vi "MTS_AutoZPos.vi"(0 "PH Dev":i32, 1 "OFlow Interv [s]":dbl, 2 "Accum Time [s]":dbl, 5 "PI System no.":i32, 11 "error in":errorcluster, 12 "Start Point":T1, 13 "Steps":i32, 14 "Step Width [um]":dbl) -> (4 "New Z":dbl, 6 "Counts":u32[](array[numeric]), 15 "error out":errorcluster)   [LabVIEW 2009]
panel:
  out "FiFo Overrun":bool
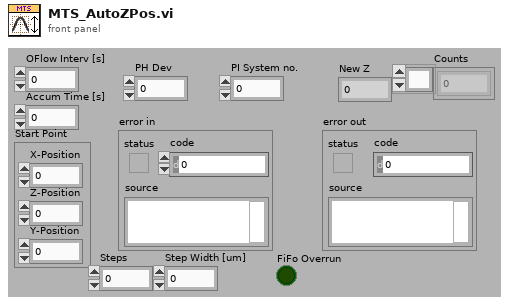
[diagram p1: front panel]
types:
  T1 = cluster{"X-Position":dbl, "Y-Position":dbl, "Z-Position":dbl}
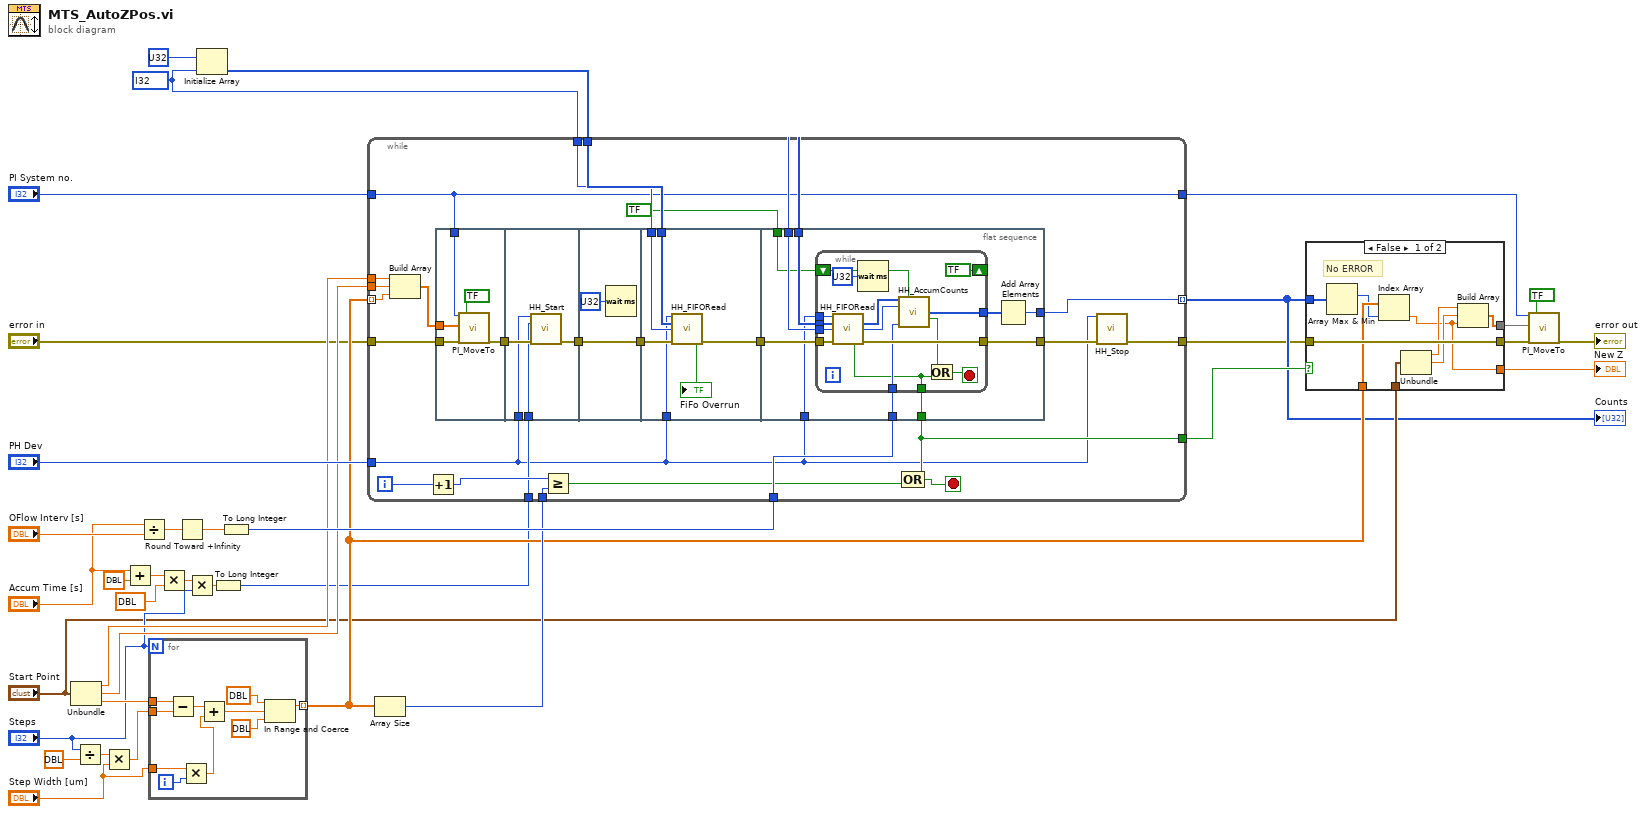
[diagram p0: block diagram]
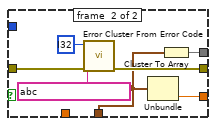
[diagram p2: hidden frame]
diagram:
  w1 = i32 ? ("dimension size")
  n1 = Unbundle("Start Point") -> ("X-Position"=w22:dbl, "Y-Position"=w23:dbl, "Z-Position"=w26:dbl)
  n2 = Divide(x="Steps", y=dbl ?) -> (x/y=w29:dbl)
  n3 = Multiply(x=w29, y="Step Width [um]") -> (x*y=w25:dbl)
  n4 = Add(x="Accum Time [s]", y=dbl ?) -> (x+y=w18:dbl)
  n5 = Divide(x="Accum Time [s]", y="OFlow Interv [s]") -> (x/y=w32:dbl)
  n6 = for {
    N: "Steps" -> [_]
    tunnel: "Step Width [um]" -> [w46]
    tunnel: w26 -> [w45]
    tunnel: w25 -> [w42]
    tunnel: [w38] -> w9 mode=indexing
    i -> [w47]
    n7 = Subtract(x=w45, y=w42) -> (x-y=w41:dbl)
    n8 = Multiply(x=w46, y=w47) -> (x*y=w40:dbl)
    n9 = Add(x=w41, y=w40) -> (x+y=w39:dbl)
    n10 = In Range and Coerce(upper limit=dbl ?, x=w39, lower limit=dbl ?) -> (coerced(x)=w38:dbl)  [unwired: 1 out]
  }
  n11 = Multiply(x=w18, y=dbl ?) -> (x*y=w16:dbl)
  n12 = Round Toward +Infinity(x=w32) -> (ceil(x): smallest int >= x=w31:dbl)
  n13 = Multiply(x=w16, y="Steps") -> (x*y=w14:dbl)
  n14 = Initialize Array(u32 ?, w1) -> (w36:u32[])
  n15 = To Long Integer(number=w14) -> (32bit integer=w3:i32)
  n16 = To Long Integer(number=w31) -> (32bit integer=w30:i32)
  n17 = Array Size(array=w9) -> (size(s)=w24:i32)
  n18 = while {
    tunnel: "error in" -> [w70]
    tunnel: w36 -> [w69]
    tunnel: w1 -> [w68]
    tunnel: "PH Dev" -> [w48]
    tunnel: [w49] -> w2
    tunnel: "PI System no." -> [w55]
    tunnel: w30 -> [w66]
    tunnel: w24 -> [w63]
    tunnel: w9 -> [w58] mode=indexing
    tunnel: w23 -> [w59]
    tunnel: w22 -> [w60]
    tunnel: [w56] -> w21
    tunnel: [w55] -> w11
    tunnel: [w54] -> w5 mode=indexing
    tunnel: w3 -> [w51]
    i -> [w65]
    stop <- w62 stop-if-true
    n19 = Build Array(w60, w59, w58) -> (w57:dbl[])
    n20 = Increment(x=w65) -> (x+1=w64:i32)
    n21 = flat-sequence {
      tunnel: w70 -> [w77]
      tunnel: [w76] -> w53
      tunnel: w55 -> [w75]
      tunnel: w57 -> [w74]
      tunnel: w53 -> [w81]
      tunnel: [w80] -> w52
      tunnel: w51 -> [w79]
      tunnel: w48 -> [w78]
      tunnel: [w82] -> w72
      tunnel: w52 -> [w82]
      tunnel: w72 -> [w89]
      tunnel: w69 -> [w88]
      tunnel: w68 -> [w87]
      tunnel: w48 -> [w86]
      tunnel: [w85] -> w71
      tunnel: w69 -> [w98]
      tunnel: w68 -> [w97]
      tunnel: w48 -> [w96]
      tunnel: [w95] -> w50
      tunnel: w71 -> [w99]
      tunnel: bool ? ("Reset") -> [w94]
      tunnel: w66 -> [w92]
      tunnel: [w91] -> w54
      tunnel: [w90] -> w56
      frame #0 {
        n22 = call "PI_MoveTo.vi"("System no."=w75, "Target position"=w74, "error in"=w77, "Move"=bool ?) -> ("error out"=w76:errorcluster)  [unwired: 13 in, 2 out]
      }
      frame #1 {
        n23 = call "HH_Start.vi"("Device Index"=w78, "Acq. Time"=w79, "error in (no error)"=w81) -> ("error out"=w80:errorcluster)  [unwired: 11 in, 1 out]
      }
      frame #2 {
        n24 = Wait (ms)(milliseconds to wait=u32 ?) -> ()  [unwired: 1 out]
      }
      frame #3 {
        n25 = call "HH_FIFORead.vi"("Device Index"=w86, "Buffer In"=w88, "Count"=w87, "error in (no error)"=w89) -> ("FiFo Overrun"=→"FiFo Overrun":bool, "error out"=w85:errorcluster)  [unwired: 7 in, 3 out]
      }
      frame #4 {
        n26 = while {
          tunnel: w99 -> [w114]
          tunnel: w98 -> [w113]
          tunnel: w97 -> [w112]
          tunnel: w96 -> [w111]
          tunnel: [w110] -> w95
          shift-right: [bool ? ("Reset")] -> _
          shift-left: w94 -> [w106]
          tunnel: [w104] -> w93
          tunnel: w92 -> [w103]
          tunnel: [w100] -> w90
          stop <- w101 stop-if-true
          n27 = call "HH_FIFORead.vi"("Device Index"=w111, "Buffer In"=w113, "Count"=w112, "error in (no error)"=w114) -> ("Buffer Out"=w108:u32[], "Data Count"=w109:i32, "FiFo Overrun"=w100:bool, "error out"=w110:errorcluster)  [unwired: 7 in, 1 out]
          n28 = Wait (ms)(milliseconds to wait=u32 ?) -> ()  [unwired: 1 out]
          n29 = call "HH_AccumCounts.vi"("Data In"=w108, "Reset"=w106, "Data Count"=w109, "Acc X Overflows"=w103) -> ("Accum Counts"=w104:u32[], "Acc Time Ok"=w102:bool)  [unwired: 7 in, 3 out]
          n30 = Or(x=w102, y=w100) -> (x .or. y?=w101:bool)
        }
        n31 = Add Array Elements(numeric array=w93) -> (sum=w91:u32)
      }
    }
    n32 = Greater Or Equal?(x=w64, y=w63) -> (x >= y?=w61:bool)
    n33 = Compound Arithmetic op=OR(w56, w61) -> (w62:bool)
    n34 = call "HH_Stop.vi"("Device Index"=w48, "error in (no error)"=w50) -> ("error out"=w49:errorcluster)  [unwired: 12 in, 1 out]
  }
  "Counts" <- w5
  n35 = case shown="False" w21 {
    tunnel: w2 -> [w123 w130]
    tunnel: [w123 w129] -> w13
    tunnel: w5 -> [w122 _]
    tunnel: w9 -> [w121 _]
    tunnel: "Start Point" -> [w119 w125]
    tunnel: [w116 w126] -> w7
    tunnel: [w115 w124] -> w6
    frame #0 {
      # "No ERROR"
      n36 = Array Max & Min(array=w122) -> (max index (indices)=w120:i32)  [unwired: 3 out]
      n37 = Index Array(array=w121, index=w120) -> (element=w115:dbl)
      n38 = Unbundle(w119) -> ("X-Position"=w118:dbl, "Y-Position"=w117:dbl)  [unwired: 1 out]
      n39 = Build Array(w118, w117, w115) -> (w116:dbl[])
    }
    frame #1 {
      n40 = call <vilib>:"Error Cluster From Error Code.vi"("error in (no error)"=w130, "error message (\"\")"=string ? ("error message (\"\")"), "error code (0)"=i32 ?) -> ("error out"=w129:errorcluster)  [unwired: 6 in]
      n41 = Unbundle(w125) -> ("Z-Position"=w124:dbl)  [unwired: 2 out]
      n42 = Cluster To Array(cluster=w125) -> (array=w126:dbl[])
    }
  }
  "New Z" <- w6
  n43 = call "PI_MoveTo.vi"("System no."=w11, "Target position"=w7, "error in"=w13, "Move"=bool ?) -> ("error out"=→"error out":errorcluster)  [unwired: 13 in, 2 out]
